vi "Add Message to Bus Controller.vi"(4 "create timestamp channel":bool, 5 "status channels directions":enum16{"Rx", "Tx", "Unspecified"}[](array[ring])=[enum."Unspecified"], 6 "parameters":T3(array[cluster]), 7 "number of words":u16, 8 "error in":errorcluster, 9 "direction":T4, 10 "name":string, 11 "port in":T1 format="%.0x") -> (0 "error out":errorcluster, 2 "message":T1=18446744073709551615 format="%.0x", 3 "port out":T1 format="%.0x")   [LabVIEW 2020, in "AIM MIL-STD-1553 Scripting.lvlib"]
uses:
  AIM MIL-STD-1553 Scripting.lvlib
  Constants.vi
  <vilib>/NI VeriStand/Custom Device API/Custom Device Item Ref.ctl
  <vilib>/NI VeriStand/Custom Device API/Custom Device API.lvlib
  Shared/Direction.ctl
  Shared/Parameter Definition.ctl
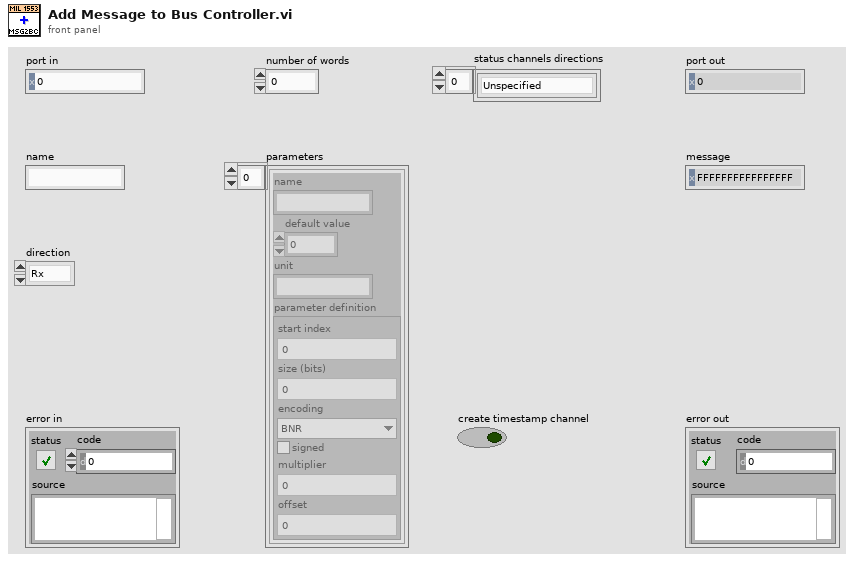
[diagram p1: front panel]
types:
  T1 = typedef "Custom Device API.lvlib/Custom Device Item Ref.ctl" = u64
  T2 = typedef "Parameter Definition.ctl" = cluster{"start index":i32, "size (bits)":i32, "encoding":enum16{"BNR", "BCD", "Discrete"}, "signed":bool, "multiplier":dbl, "offset":dbl}
  T3 = cluster{"name":string, "default value":dbl, "unit":string, "parameter definition":T2}[]
  T4 = typedef "Direction.ctl" = enum16{"Rx", "Tx"}
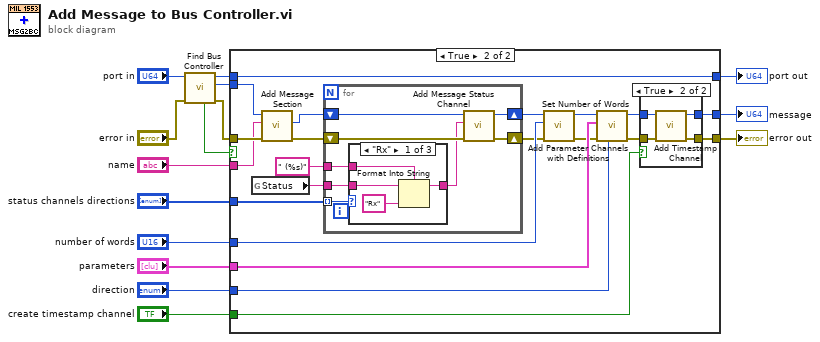
[diagram p0: block diagram]
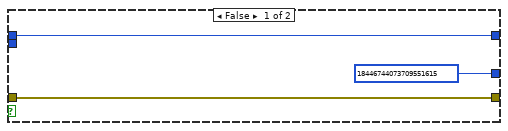
[diagram p2: hidden frame]
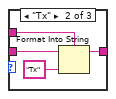
[diagram p3: hidden frame]
diagram:
  n1 = call "Find Bus Controller.vi"("error in"="error in", "port in"="port in") -> ("error out"=w7:errorcluster, "bus controller"=w6:T1, "port out"=w5:T1, "found?"=w4:bool)  [unwired: 6 in]
  n2 = case shown="True" w4 {
    tunnel: w5 -> [w18 w30]
    tunnel: w6 -> [_ w38]
    tunnel: w7 -> [w17 w39]
    tunnel: [w17 w28] -> w8
    tunnel: [w18 w30] -> w9
    tunnel: "number of words" -> [_ w37]
    tunnel: "parameters" -> [_ w36]
    tunnel: "name" -> [_ w33]
    tunnel: "direction" -> [_ w32]
    tunnel: "create timestamp channel" -> [_ w31]
    tunnel: "status channels directions" -> [_ w21]
    tunnel: [T1 18446744073709551615 ("message out") w26] -> w1
    frame False {
    }
    frame True {
      n3 = global read "Constants.vi" "Status"() -> (w20:string)
      n4 = call "Add Message Section.vi"("error in"=w39, "message name"=w33, "bus controller in"=w38) -> ("error out"=w25:errorcluster, "message"=w24:T1)  [unwired: 6 in, 1 out]
      n5 = for {
        shift-right: [w44] -> w23
        shift-left: w25 -> [w46]
        shift-right: [w45] -> w22
        shift-left: w24 -> [w47]
        tunnel: w21 -> [w43] mode=indexing
        tunnel: w20 -> [w42]
        tunnel: " (%s)" ("format string") -> [w40]
        n6 = case shown="\"Rx\"" w43 {
          tunnel: w42 -> [w51 w55 w56]
          tunnel: [w49 w53 w56] -> w41
          tunnel: w40 -> [w50 w54 _]
          frame "Rx" {
            n7 = Format Into String(format string=w50, initial string=w51, "Rx" ("Status")) -> (resulting string=w49:string)  [unwired: 1 in, 1 out]
          }
          frame "Tx" {
            n8 = Format Into String(format string=w54, initial string=w55, "Tx" ("Status")) -> (resulting string=w53:string)  [unwired: 1 in, 1 out]
          }
          frame Default {
          }
        }
        n9 = call "Add Message Status Channel.vi"("error in"=w46, "name (empty = \"Status\")"=w41, "message in"=w47) -> ("error out"=w44:errorcluster, "message out"=w45:T1)  [unwired: 6 in, 1 out]
      }
      n10 = call "Set Number of Words.vi"("error in"=w23, "number of words"=w37, "message in"=w22) -> ("error out"=w34:errorcluster, "message out"=w35:T1)  [unwired: 7 in]
      n11 = call "Add Parameter Channels with Definitions.vi"("direction"=w32, "error in"=w34, "parameters"=w36, "message in"=w35) -> ("error out"=w29:errorcluster, "message out"=w27:T1)  [unwired: 6 in]
      n12 = case shown="True" w31 {
        tunnel: w29 -> [w58 w62]
        tunnel: w27 -> [w57 w61]
        tunnel: [w58 w60] -> w28
        tunnel: [w57 w59] -> w26
        frame False {
        }
        frame True {
          n13 = call "Add Timestamp Channel.vi"("error in"=w62, "message section in"=w61) -> ("error out"=w60:errorcluster, "message section out"=w59:T1)  [unwired: 7 in, 1 out]
        }
      }
    }
  }
  "port out" <- w9
  "error out" <- w8
  "message" <- w1
